vi "Global Variables PID.vi"() -> ()   [LabVIEW 2012]
panel:
  in  "PV (i-1)":dbl format="%.3g"
  in  "Integral (i-1)":dbl format="%.3g"
  in  "Error (i-1)":dbl format="%.3g"
  # "This is a list of Variables in the Custom PID v1_1.vi. It is used to transfer data output of the subVI for the next iteration. This cleans the PID subVI by eliminating wire clutter."
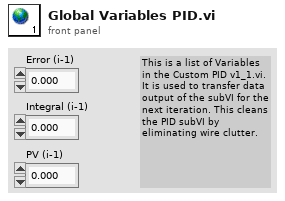
[diagram p1: front panel]
diagram:
